vi "CSConnectGUI.EmergencyOff.vi"(0 "i ref in":refnum<vi>, 5 "error in (no error)":errorcluster) -> (14 "i ref out":refnum<vi>, 19 "error out":errorcluster)   [LabVIEW 2014, in "CSConnectGUI.lvlib"]
doc: "Performs an emergency OFF of the power supply, even bypassing the GOG."
uses:
  CSConnectGUI.lvlib
  CSCore/BaseProcess/BaseProcess.lvlib
  CSCore/GUIs/GOGUserGUIs/DeviceBaseGUI/DeviceBaseGUI.lvlib
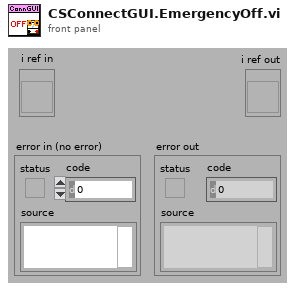
[diagram p1: front panel]
types:
  T1 = typedef "DeviceBaseGUI.lvlib/DeviceBaseGUI.i attribute.ctl" = cluster{"GOGFrontPanel.i attribute":T2}
  T2 = typedef "GOGFrontPanel.lvlib/GOGFrontPanel.i attribute.ctl" = cluster{"GOGObject":string, "Object":string, "Method":string, "Descriptor":T3, "Input Descriptor":string, "Output Descriptor":string, "inputNames":string[], "outputNames":string[], "Values":cluster{"descriptor":string, "value":string}[]}
  T3 = typedef "BaseProcess.lvlib/BaseProcess.descriptor string definition.ctl" = string
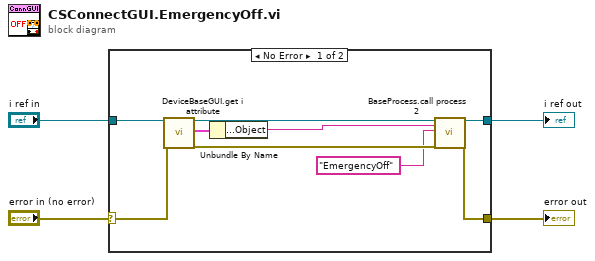
[diagram p0: block diagram]
diagram:
  n1 = case shown="No Error" "error in (no error)" {
    selector: "error in (no error)" -> [w12 w14]
    tunnel: [w7 w15] -> w4
    tunnel: [w8 w14] -> w3
    tunnel: "i ref in" -> [w13 w15]
    frame No Error {
      n2 = call "DeviceBaseGUI.get i attribute.vi"("i ref in"=w13, "error in (no error)"=w12) -> ("i ref out"=w10:refnum<vi>, "i attribute"=w11:T1, "error out"=w9:errorcluster)  [unwired: 15 in]
      n3 = Unbundle By Name(w11) -> ("GOGFrontPanel.i attribute.Object"=w6:string)
      n4 = call "BaseProcess.call process 2.vi"("i ref in"=w10, "Object"=w6, "Selector"="EmergencyOff", "error in (no error)"=w9) -> ("i ref out"=w7:refnum<vi>, "error out"=w8:errorcluster)  [unwired: 14 in]
    }
    frame Error {
    }
  }
  "error out" <- w3
  "i ref out" <- w4
